vi "CoreLoop.vi"(8 "error in":errorcluster, 11 "CONTROLLER in":refnum<class "CONTROLLER.lvclass">) -> (0 "error out":errorcluster, 3 "CONTROLLER out":refnum<class "CONTROLLER.lvclass">)   [LabVIEW 2013, in "CONTROLLER.lvclass"]
uses:
  CONTROLLER.lvclass
  CONTROLLER.lvclass/CONTROLLER.ctl
  View/base/VIEW.lvclass
panel:
  in  "Stop":bool
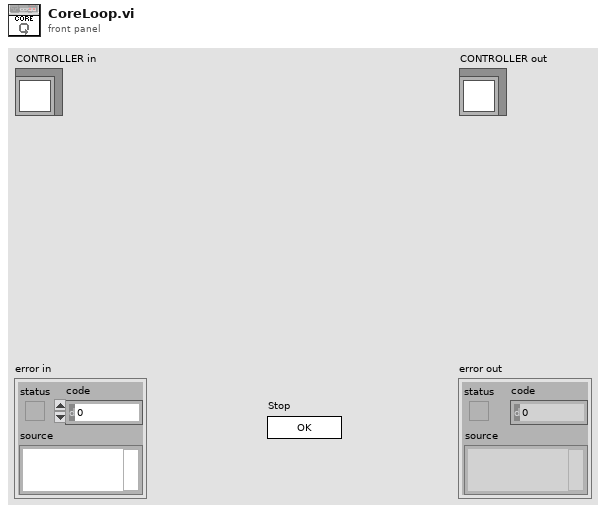
[diagram p1: front panel]
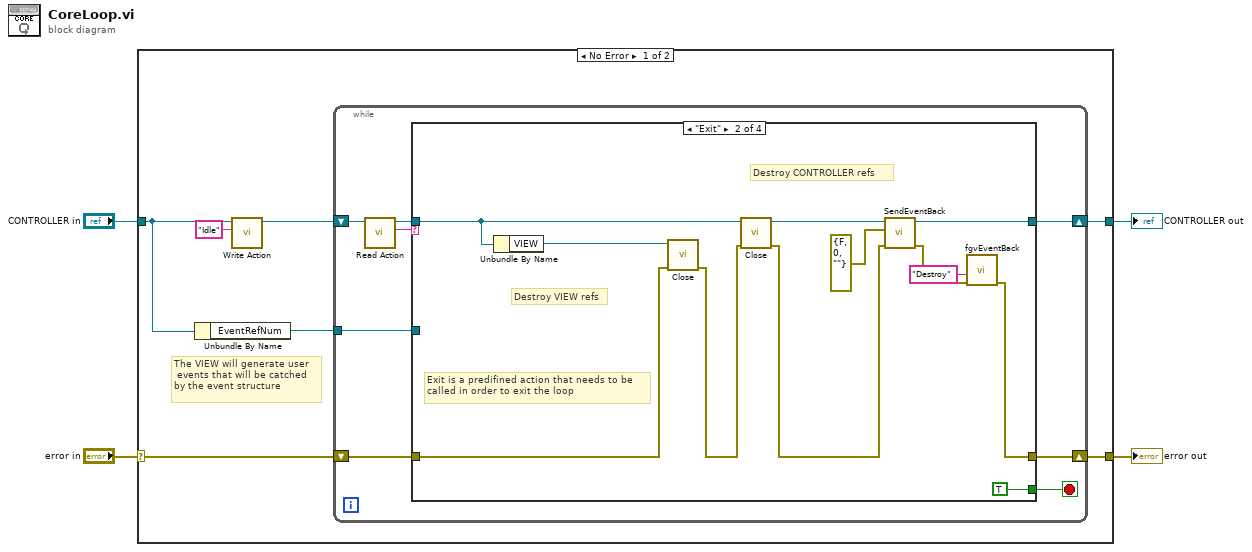
[diagram p0: block diagram]
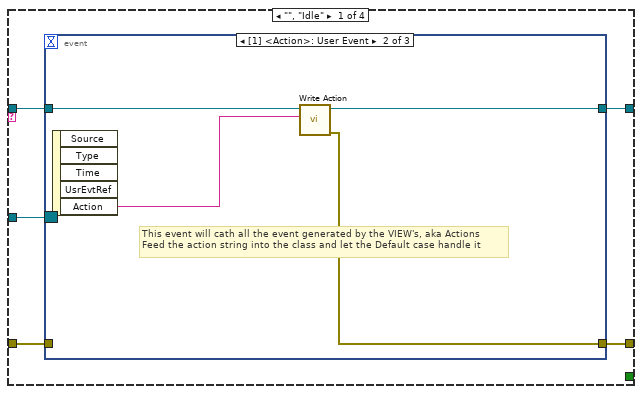
[diagram p2: hidden frame]
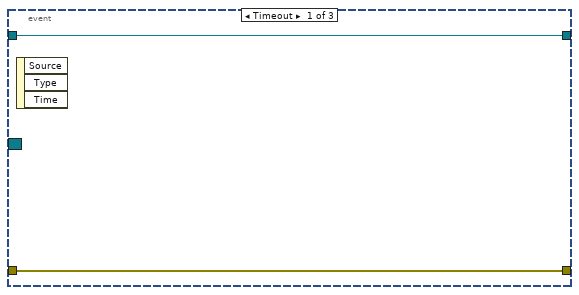
[diagram p3: hidden frame]
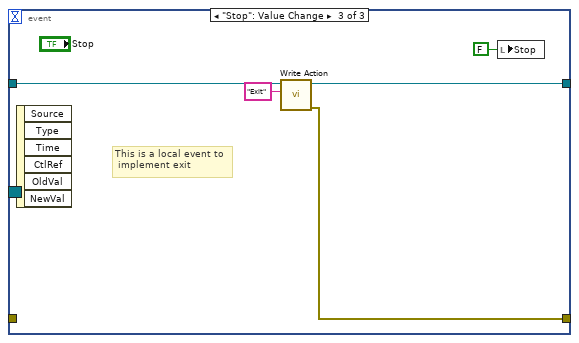
[diagram p4: hidden frame]
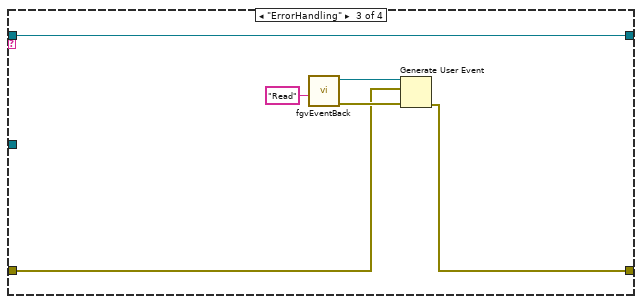
[diagram p5: hidden frame]
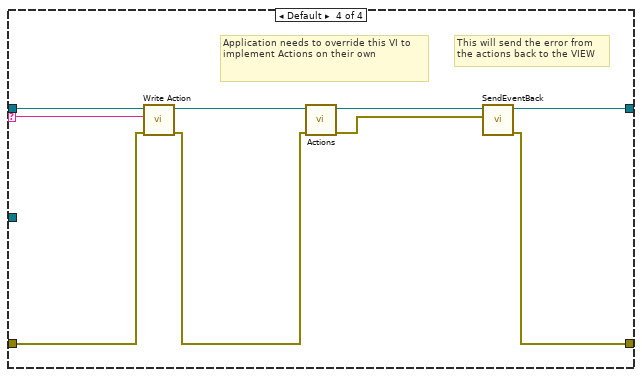
[diagram p6: hidden frame]
diagram:
  n1 = case shown="No Error" "error in" {
    selector: "error in" -> [w9 w64]
    tunnel: [w11 w64] -> w3
    tunnel: [w10 w63] -> w1
    tunnel: "CONTROLLER in" -> [w6 w63]
    frame No Error {
      # "The VIEW will generate user\n events that will be catched \nby the event structure"
      n2 = Unbundle By Name(w6) -> ("EventRefNum"=w5:refnum<event-registration>)
      n3 = call-dynamic "Write Action.vi"("Action"="Idle", "CONTROLLER in"=w6) -> ("CONTROLLER out"=w8:refnum<class "CONTROLLER.lvclass">)  [unwired: 8 in, 1 out]
      n4 = while {
        shift-right: [w19] -> w10
        shift-left: w8 -> [w18]
        shift-right: [w14] -> w11
        shift-left: w9 -> [w12]
        tunnel: w5 -> [w13]
        stop <- w15 stop-if-true
        n5 = call-dynamic "Read Action.vi"("CONTROLLER in"=w18) -> ("Action"=w16:string, "CONTROLLER out"=w17:refnum<class "CONTROLLER.lvclass">)  [unwired: 8 in, 1 out]
        n6 = case shown="\"Exit\"" w16 {
          selector: w16 -> [_ _ _ w60]
          tunnel: w17 -> [w20 w45 w53 w62]
          tunnel: [w21 w41 w53 w56] -> w19
          tunnel: [_ TRUE _ _] -> w15
          tunnel: [w23 w37 w48 w54] -> w14
          tunnel: w12 -> [w22 w46 w49 w59]
          tunnel: w13 -> [w24 _ _ _]
          frame "", "Idle" {
            n7 = event shown="[1] <Action>: User Event" {
              selector: w24 -> [_ _ _]
              dyn-events: _ -> [_ _ _]
              timeout: _ -> [_ _ _]
              tunnel: [w26 w27 w32] -> w23
              tunnel: w22 -> [w26 _ _]
              tunnel: [w25 w29 w34] -> w21
              tunnel: w20 -> [w25 w30 w35]
              event Timeout {
                n8 = event-data() -> ()  [unwired: 1 in, 3 out]
              }
              event User Event {
                # "This event will cath all the event generated by the VIEW's, aka Actions\nFeed the action string into the class and let the Default case handle it"
                n9 = event-data() -> ("Action"=w28:string)  [unwired: 1 in, 4 out]
                n10 = call-dynamic "Write Action.vi"("Action"=w28, "CONTROLLER in"=w30) -> ("error out"=w27:errorcluster, "CONTROLLER out"=w29:refnum<class "CONTROLLER.lvclass">)  [unwired: 8 in]
              }
              event "Stop": Value Change {
                # "This is a local event to\n implement exit"
                n11 = event-data() -> ()  [unwired: 1 in, 6 out]
                n12 = call-dynamic "Write Action.vi"("Action"="Exit", "CONTROLLER in"=w35) -> ("error out"=w32:errorcluster, "CONTROLLER out"=w34:refnum<class "CONTROLLER.lvclass">)  [unwired: 8 in]
                n13 = local write "Stop"(FALSE ("Stop")) -> ()
              }
            }
          }
          frame "Exit" {
            # "Destroy CONTROLLER refs"
            # "Destroy VIEW refs"
            # "Exit is a predifined action that needs to be \ncalled in order to exit the loop"
            n14 = Unbundle By Name(w45) -> ("VIEW"=w44:refnum<class "VIEW.lvclass">)
            n15 = call-dynamic "Close.vi"("error in (no error)"=w46, "VIEW in"=w44) -> ("error out"=w42:errorcluster)  [unwired: 8 in, 1 out]
            n16 = call-dynamic "Close.vi"("error in (no error)"=w42, "CONTROLLER in"=w45) -> ("error out"=w40:errorcluster, "CONTROLLER out"=w43:refnum<class "CONTROLLER.lvclass">)  [unwired: 8 in]
            n17 = call "SendEventBack.vi"("error in"=w40, "error VIEW"=errorcluster {"status"=FALSE, "code"=0, "source"=""}, "CONTROLLER in"=w43) -> ("error out"=w38:errorcluster, "CONTROLLER out"=w41:refnum<class "CONTROLLER.lvclass">)  [unwired: 7 in]
            n18 = call "fgvEventBack.vi"("error in (no error)"=w38, "Cmd"="Destroy") -> ("error out"=w37:errorcluster)  [unwired: 7 in, 2 out]
          }
          frame "ErrorHandling" {
            n19 = call "fgvEventBack.vi"("Cmd"="Read") -> ("error out"=w50:errorcluster, "EventData out"=w51:refnum<user-event>)  [unwired: 8 in, 1 out]
            n20 = Generate User Event(user event=w51, event data cluster=w49, error in=w50) -> (error out=w48:errorcluster)  [unwired: 1 in, 1 out]
          }
          frame Default {
            # "This will send the error from \nthe actions back to the VIEW"
            # "Application needs to override this VI to\nimplement Actions on their own"
            n21 = call-dynamic "Write Action.vi"("error in (no error)"=w59, "Action"=w60, "CONTROLLER in"=w62) -> ("error out"=w58:errorcluster, "CONTROLLER out"=w61:refnum<class "CONTROLLER.lvclass">)  [unwired: 7 in]
            n22 = call-dynamic "Actions.vi"("error in (no error)"=w58, "CONTROLLER in"=w61) -> ("error out"=w55:errorcluster, "CONTROLLER out"=w57:refnum<class "CONTROLLER.lvclass">)  [unwired: 8 in]
            n23 = call "SendEventBack.vi"("error VIEW"=w55, "CONTROLLER in"=w57) -> ("error out"=w54:errorcluster, "CONTROLLER out"=w56:refnum<class "CONTROLLER.lvclass">)  [unwired: 8 in]
          }
        }
      }
    }
    frame Error {
    }
  }
  "error out" <- w3
  "CONTROLLER out" <- w1
